vi "get published streams.vi"(8 "error in":errorcluster, 11 "engine configuration in":refnum<class "engine configuration.lvclass">) -> (0 "error out":errorcluster, 2 "published streams":T1[](array[typedef]), 3 "engine configuration out":refnum<class "engine configuration.lvclass">)   [LabVIEW 2013, in "engine configuration.lvclass"]
uses:
  engine configuration.lvclass
  unique channel identifier.ctl
  engine configuration.lvclass/engine configuration.ctl
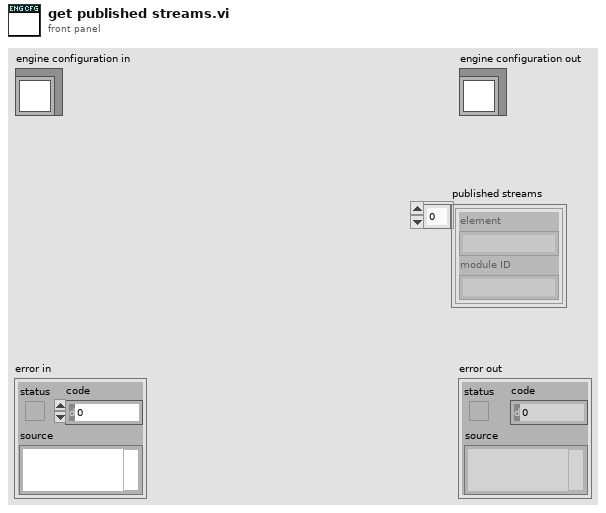
[diagram p1: front panel]
types:
  T1 = typedef "engine configuration.lvclass/unique channel identifier.ctl" = cluster{"element":string, "module ID":string}
  T2 = typedef "engine configuration.lvclass/simple mapping.ctl" = cluster{"module ID":string[], "publisher":string[], "subscribers":T3[]}
  T3 = typedef "engine configuration.lvclass/module channel pairings.ctl" = cluster{"modules":string[], "element":string[]}
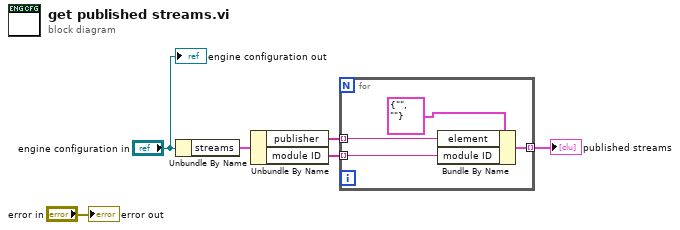
[diagram p0: block diagram]
diagram:
  n1 = Unbundle By Name("engine configuration in") -> ("streams"=w4:T2)
  n2 = Unbundle By Name(w4) -> ("publisher"=w3:string[], "module ID"=w2:string[])
  n3 = for {
    tunnel: w3 -> [w9] mode=indexing
    tunnel: w2 -> [w8] mode=indexing
    tunnel: [w7] -> w1 mode=indexing
    n4 = Bundle By Name(cluster=T1 {"element"="", "module ID"=""} ("unique channel identifier"), "element"=w9, "module ID"=w8) -> (w7:T1)
  }
  "published streams" <- w1
  "error out" <- "error in"
  "engine configuration out" <- "engine configuration in"
